vi "Async.Engine.Close.vi"(8 "error in (no error)":errorcluster, 11 "Async in":refnum<class "VS Inline Async API.lvclass">) -> (0 "error out":errorcluster, 3 "Async out":refnum<class "VS Inline Async API.lvclass">)   [LabVIEW 2015, in "VS Inline Async API.lvlib" / "VS Inline Async API.lvclass"]
uses:
  VS Inline Async API.lvclass
  VS Inline Async API.lvclass/VS Inline Async API.ctl
  _Data Access Engine/Data Access Engine/Data Access Engine.lvclass
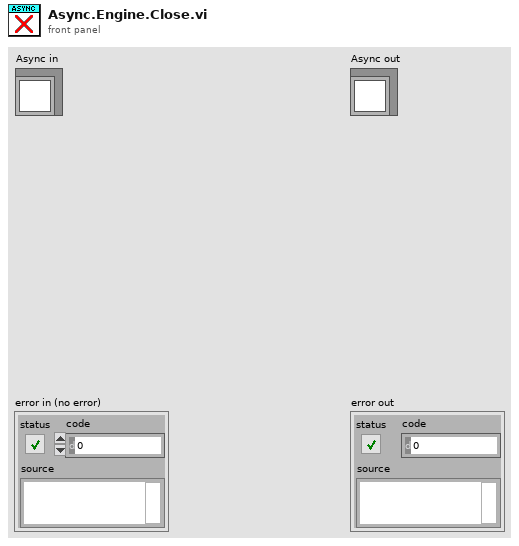
[diagram p1: front panel]
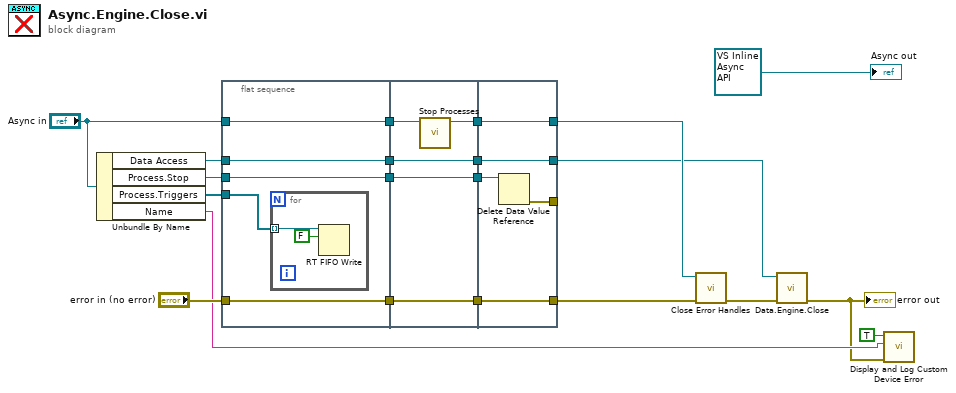
[diagram p0: block diagram]
diagram:
  n1 = Unbundle By Name("Async in") -> ("Data Access"=w6:refnum<class "Data Access Engine.lvclass">, "Process.Stop"=w14:refnum<data-value>, "Process.Triggers"=w5:refnum<k33>[], "Name"=w16:string)
  n2 = flat-sequence {
    tunnel: [w26] -> w21
    tunnel: "error in (no error)" -> [w26]
    tunnel: [w25] -> w15
    tunnel: "Async in" -> [w25]
    tunnel: w14 -> [w24]
    tunnel: [w24] -> w13
    tunnel: [w23] -> w7
    tunnel: w6 -> [w23]
    tunnel: w5 -> [w22]
    tunnel: [w33] -> w4
    tunnel: w21 -> [w33]
    tunnel: w15 -> [w32]
    tunnel: [w31] -> w3
    tunnel: w13 -> [w31]
    tunnel: [w30] -> w2
    tunnel: [w29] -> w1
    tunnel: w7 -> [w29]
    tunnel: [w38] -> w19
    tunnel: w4 -> [w38]
    tunnel: w3 -> [w37]
    tunnel: [w36] -> w11
    tunnel: w2 -> [w36]
    tunnel: [w35] -> _
    tunnel: [w34] -> w8
    tunnel: w1 -> [w34]
    frame #0 {
      n3 = for {
        tunnel: w22 -> [w28] mode=indexing
        n4 = RT FIFO Write(0:w28, 1:FALSE ("element")) -> ()  [unwired: 3 in, 4 out]
      }
    }
    frame #1 {
      n5 = call "Stop Processes.vi"("VS Inline Async API in"=w32) -> ("VS Inline Async API out"=w30:refnum<class "VS Inline Async API.lvclass">)  [unwired: 10 in]
    }
    frame #2 {
      n6 = Delete Data Value Reference(data value reference=w37) -> (error out=w35:errorcluster)  [unwired: 1 in, 1 out]
    }
  }
  n7 = call "Close Error Handles.vi"("error in"=w19, "Async in"=w11) -> ("error out"=w10:errorcluster)  [unwired: 8 in, 1 out]
  n8 = call "Data.Engine.Close.vi"("error in (no error)"=w10, "Data Access API in"=w8) -> ("error out"=w9:errorcluster)  [unwired: 8 in, 1 out]
  "error out" <- w9
  n9 = call "Display and Log Custom Device Error.vi"("error out"=w9, "Your code's public name"=w16, "Custom Device? (T)"=TRUE) -> ()  [unwired: 9 in]
  "Async out" <- refnum<class "VS Inline Async API.lvclass"> refnum ("Async out")
